vi "Sweep_AIWFM_time.vi"(8 "error in (no error)":errorcluster, 11 "Transport":refnum<class "SMO.Transport.lvclass">) -> (0 "error out":errorcluster, 3 "Transport.lvclass":refnum<class "SMO.Transport.lvclass">)   [LabVIEW 2019, in "SMO.Transport.lvclass"]
uses:
  SMO.Transport.lvclass
  <userlib>/LevyLab/Instrument Framework/Instrument Types/Cryostat/Instrument.Cryostat.lvclass
  SMO.Control Experiment/SMO.Control Experiment.lvclass
  <userlib>/LevyLab/Lockin-Multichannel/Instrument.Lockin/Instrument.Lockin.lvclass
  <userlib>/LevyLab/Krohn Hite 7008/Instrument.KH7008.lvclass
  SMO.Control Experiment/Private/Control Experiment SM/Typedefs/Instruments--cluster.ctl
  <userlib>/LevyLab/Instrument Framework/Instrument Types/VSource/Instrument.VSource.lvclass
  <userlib>/LevyLab/Instrument Framework/Instrument Types/VNA/Instrument.VNA.lvclass
  <userlib>/LevyLab/Instrument Framework/Instrument Types/Strain/Instrument.Strain.lvclass
  <userlib>/LevyLab/Instrument Framework/Instrument Types/CBridge/Instrument.CBridge.lvclass
  <vilib>/Waveform/WDTOps.llb/WDT Append Waveforms DBL.vi
  <userlib>/LevyLab/XY Utilities/xy_utilities.lvlib
  <userlib>/LevyLab/XY Utilities/subVIs/Waveform to XY (single).vi
  <userlib>/LevyLab/XY Utilities/subVIs/Get X and Y (single).vi
  <userlib>/LevyLab/Lockin-Multichannel/Lockin.DAQ/Typedefs/State-enum.ctl
  <userlib>/LevyLab/Lockin-Multichannel/Lockin.DAQ/Typedefs/Sweep Configuration--Cluster.ctl
  <userlib>/LevyLab/Lockin-Multichannel/Lockin.DAQ/Typedefs/Sweep Pattern--Enum.ctl
  <userlib>/LevyLab/Lockin-Multichannel/Instrument.Lockinl.UI/Typedefs/Sweep Channel--Cluster.ctl
  <userlib>/LevyLab/Instrument Framework/Instrument Types/Delay Line/Instrument.DelayLine.lvclass
panel:
  out "elapsed time (s)":u32=36594
  out "time b/w points (ms)":u32=533
  in  "Stop":bool
  in  "Tab Control":enum32{"Control", "Waveform", "Other"}(tab)
  in  "Sweep Time (s)":dbl=10.0 format="%#_3p"
  in  "Initial Wait (s)":u32=1
  in  "Return to Start":bool=TRUE
  in  "wait (ms)":u32=500
  in  "Experiment Description":string="SA40321H:\nT=80mK, BG=0V, B=-9T\nLoop 0: sgR: -1V to 1V, 20mV step\nInner loop: I+/I-: 28/2   -180mV to 220mV, sweep time 10s\nsgL (lead 1): 0V\nsgR (lead 3): sweep\n    \nI+/I-: 28/2   -180mV to 220mV, sweep time 10s\nV+/V-: 5/2\nsgL-lead 1; sgR-lead 3\n\ntc: 100ms\norder: 4\n\n"
  in  "Experiment Folder":string="01-sgR IV for RD"
  in  "Channels":T1[](array[typedef]) {"Channel" items=["AO1"=1, "AO2"=2]; "Start" format="%#_6p"; "End" format="%#_6p"}
  out "AO":waveform(dbl)(graph)={"t0"=timestamp(3666661573.979815 s since 1904-01-01), "dt"=0.0009999999996825864, "Y"=array[14000 elements]}
  out "AI vs AO":cluster{"Y":dbl[], "Y":dbl[]}[](graph)
  out "AI":waveform(dbl)[](graph)=[{"t0"=timestamp(3666661571.9305677 s since 1904-01-01), "dt"=0.0009999999996825864, "Y"=array[14000 elements], "attributes"=variant("NI_ChannelName"=variant(string "Dev1/ai0"), "NI_UnitDescription"=variant(string "Volts"))}, {"t0"=timestamp(3666661571.9305677 s since 1904-01-01), "dt"=0.0009999999996825864, "Y"=array[14000 elements], "attributes"=variant("NI_ChannelName"=variant(string "Dev1/ai1"), "NI_UnitDescription"=variant(string "Volts"))}, {"t0"=timestamp(3666661571.9305677 s since 1904-01-01), "dt"=0.0009999999996825864, "Y"=array[14000 elements], "attributes"=variant("NI_ChannelName"=variant(string "PXI1Slot8/ai0"), "NI_UnitDescription"=variant(string "Volts"))}, {"t0"=timestamp(3666661571.9305677 s since 1904-01-01), "dt"=0.0009999999996825864, "Y"=array[14000 elements], "attributes"=variant("NI_ChannelName"=variant(string "PXI1Slot8/ai1"), "NI_UnitDescription"=variant(string "Volts"))}, {"t0"=timestamp(3666661569.527568 s since 1904-01-01), "dt"=0.0009999999996825864, "Y"=array[14000 elements], "attributes"=variant("NI_ChannelName"=variant(string "Dev2/ai0"), "NI_UnitDescription"=variant(string "Volts"))}, {"t0"=timestamp(3666661569.527568 s since 1904-01-01), "dt"=0.0009999999996825864, "Y"=array[14000 elements], "attributes"=variant("NI_ChannelName"=variant(string "Dev2/ai1"), "NI_UnitDescription"=variant(string "Volts"))}]
  out "Status":T3
  out "Current State":string="File: Save"
  # "*** These controls are only read if this VI is the top level. If is is called from Sweep Control then the folder and comments come from Sweep Control.vi ***"
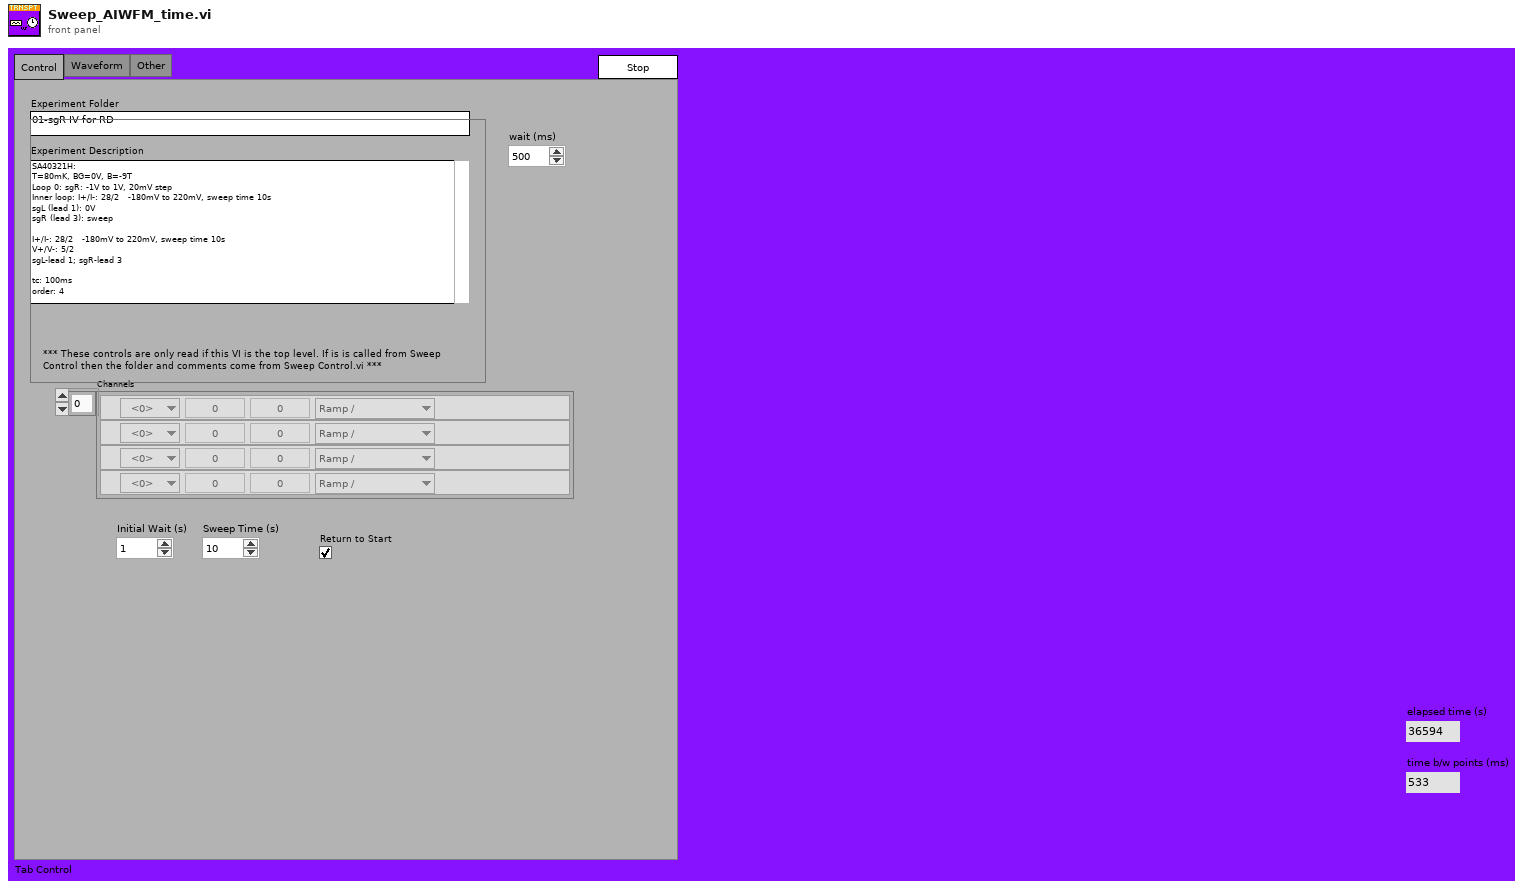
[diagram p1: front panel]
types:
  T1 = typedef "Instrument.Lockin.UI.lvclass/Sweep Channel--Cluster.ctl" = cluster{"End":dbl, "Start":dbl, "Channel":u16, "Pattern":T2}
  T2 = typedef "Lockin.DAQ.lvclass/Sweep Pattern--Enum.ctl" = enum16{"Ramp /", "Ramp /\\", "Smooth Ramp _/", "Smooth Ramp _/\\_", "Frequency"}
  T3 = typedef "Lockin.DAQ.lvclass/State-enum.ctl" = enum16{"idle", "created", "started", "stopped", "sweeping"}
  T4 = enum32{"Invalid", "Standard", "Closed", "Hidden", "Minimized", "Maximized"}
  T5 = enum32{"invalid app kind", "Development System", "Run Time System", "Student Edition", "Embedded LabVIEW", "Evaluation", "Custom"}
  T6 = typedef "SMO.Control Experiment.lvclass/Instruments--cluster.ctl" = cluster{"Lockin":refnum<class "Instrument.Lockin.lvclass">, "Temperature":refnum<class "Instrument.Cryostat.lvclass">, "Magnet":refnum<class "Instrument.Cryostat.lvclass">, "Rotator":refnum<class "Instrument.Cryostat.lvclass">, "Level":refnum<class "Instrument.Cryostat.lvclass">, "C Bridge":refnum<class "Instrument.CBridge.lvclass">, "Optical Delay Line":refnum<class "Instrument.DelayLine.lvclass">, "Strain Cell":refnum<class "Instrument.Strain.lvclass">, "VNA":refnum<class "Instrument.VNA.lvclass">, "Voltage Source":refnum<class "Instrument.VSource.lvclass">, "KH7008":refnum<class "Instrument.KH7008.lvclass">[]}
  T7 = typedef "Lockin.DAQ.lvclass/Sweep Configuration--Cluster.ctl" = cluster{"Sweep Time (s)":dbl, "Initial Wait (s)":dbl, "Return to Start":bool, "Channels":T1[]}
  T8 = cluster{"Core":cluster{"Current VI Reference":refnum<vi>, "Close Panel on Exit?":bool}, "Transport":refnum<class "SMO.Transport.lvclass">, "Control Experiment":refnum<class "SMO.Control Experiment.lvclass">, "Notifier":refnum<notifier>, "Instruments":T6, "path":path, "time":dbl, "temperature":dbl, "magnet field":dbl, "AI XY (new)":cluster{dbl[], dbl[]}[], "AI XY (all)":cluster{dbl[], dbl[]}[], "AI Waveform (s)":waveform(dbl)[], "t0":timestamp, "ms [0]":u32, "ms [i]":u32, "AO Waveform (s)":waveform(dbl)[], "Execution:State":enum32{"Bad", "Idle", "Run top level", "Running"}}
  T9 = enum32{"Bad", "Idle", "Run top level", "Running"}
  T10 = cluster{"Current VI Reference":refnum<vi>, "Close Panel on Exit?":bool}
  T11 = typedef "Instrument.DAQ.lvclass/Get State-enum.ctl" = enum16{"idle", "created", "started", "stopped", "sweeping"}
  T12 = typedef "Instrument.DAQ.lvclass/AO.Channel--Cluster--Array.ctl" = T13[]
  T13 = typedef "Instrument.DAQ.lvclass/AO.Channel--Cluster.ctl" = cluster{"Enable?":bool, "Channel":i32, "Amplitude":dbl, "Offset":dbl, "Frequency":dbl, "Phase":dbl, "Function":T14, "Sweeping?":bool}
  T14 = typedef "Instrument.DAQ.lvclass/AO.Channel.Function--Enum.ctl" = enum16{"Sine", "Triangle", "Square"}
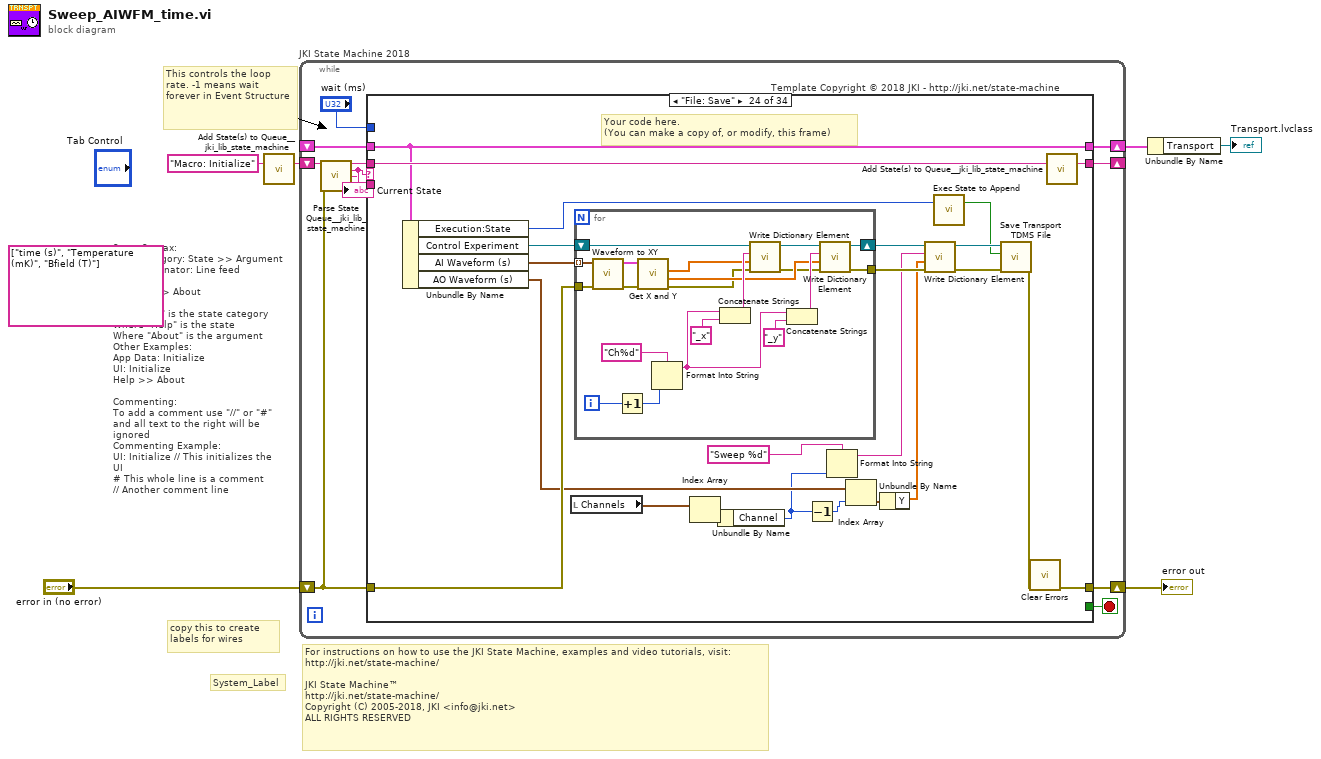
[diagram p0: block diagram]
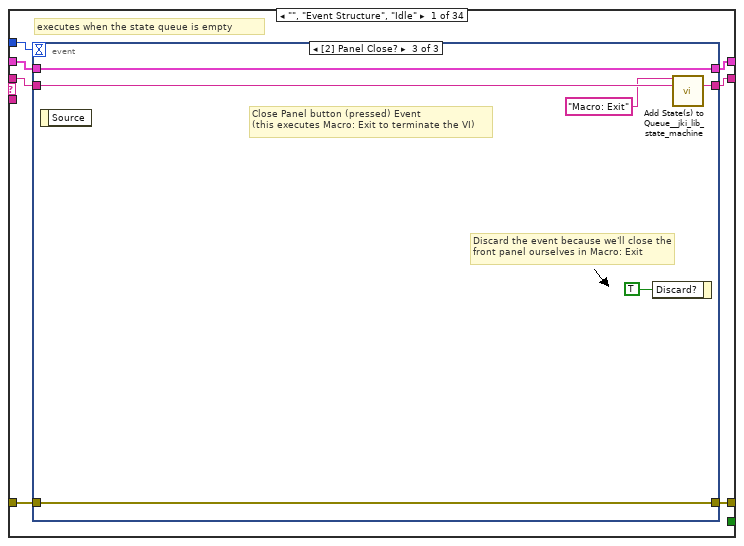
[diagram p2: hidden frame]
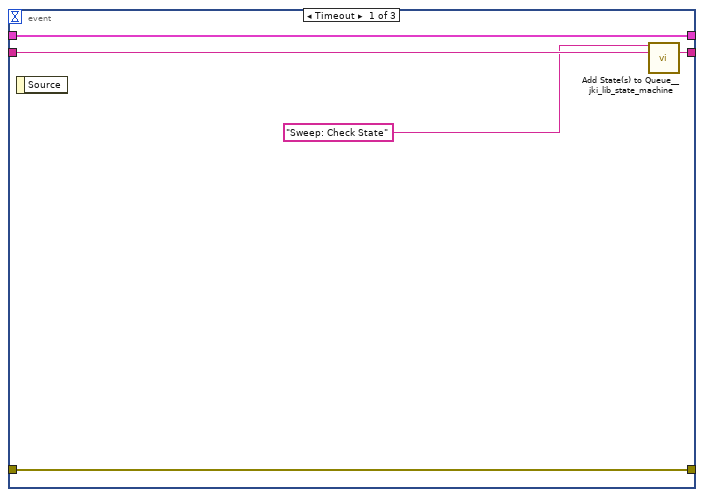
[diagram p3: hidden frame]
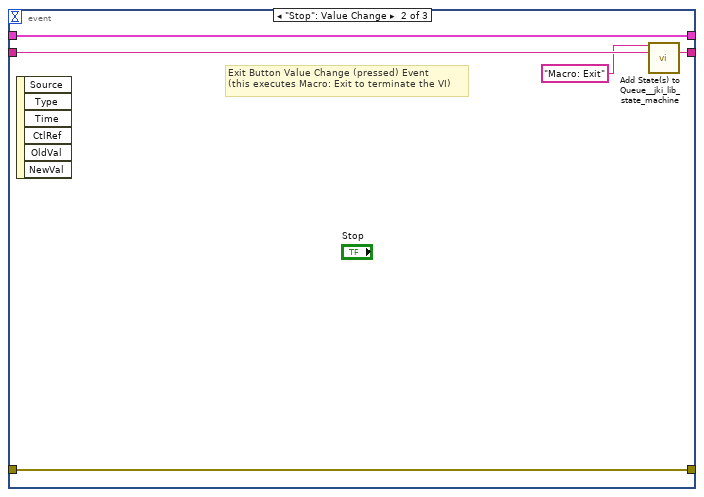
[diagram p4: hidden frame]
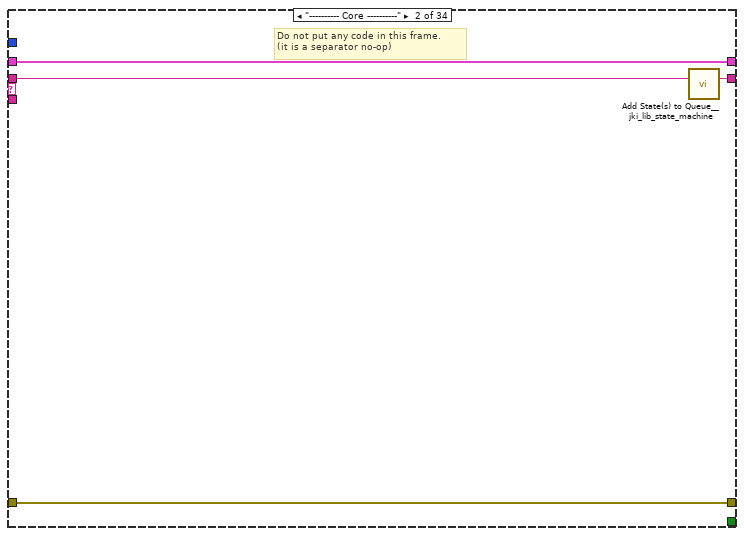
[diagram p5: hidden frame]
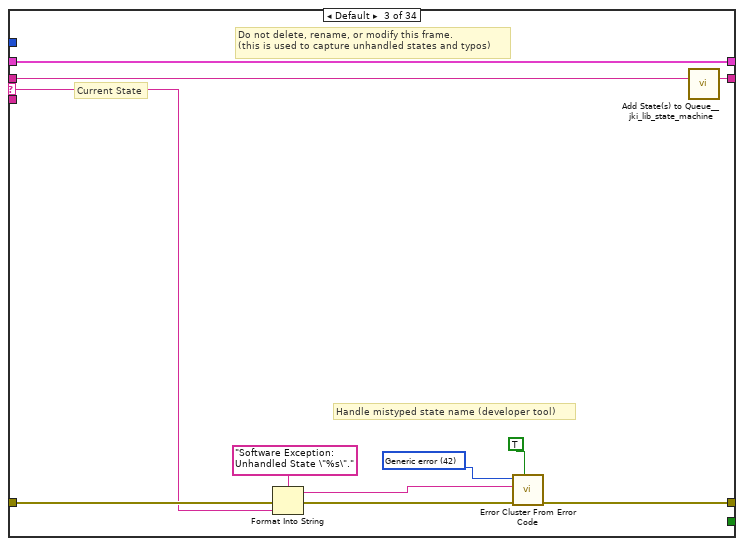
[diagram p6: hidden frame]
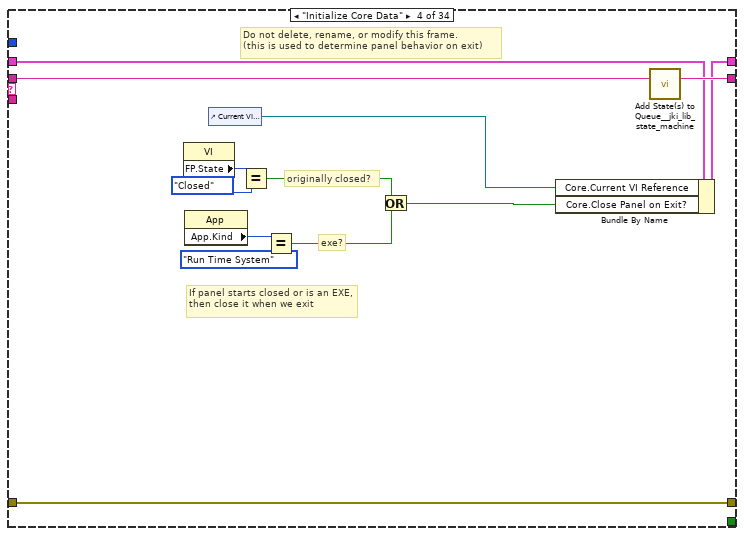
[diagram p7: hidden frame]
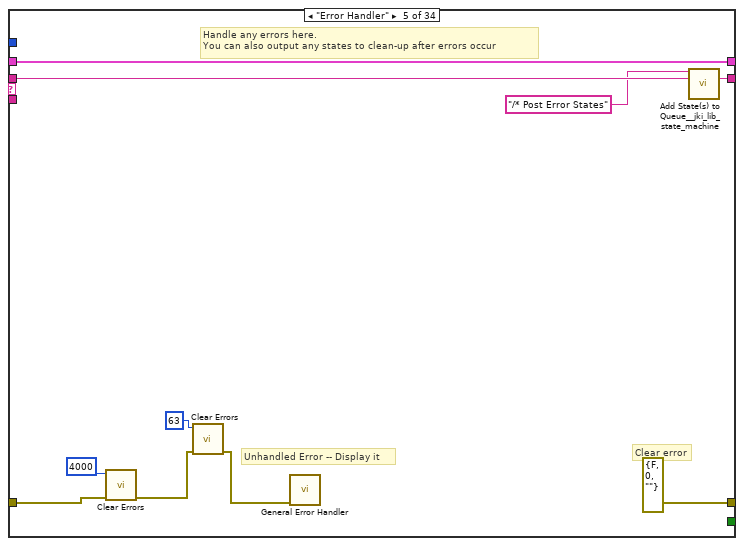
[diagram p8: hidden frame]
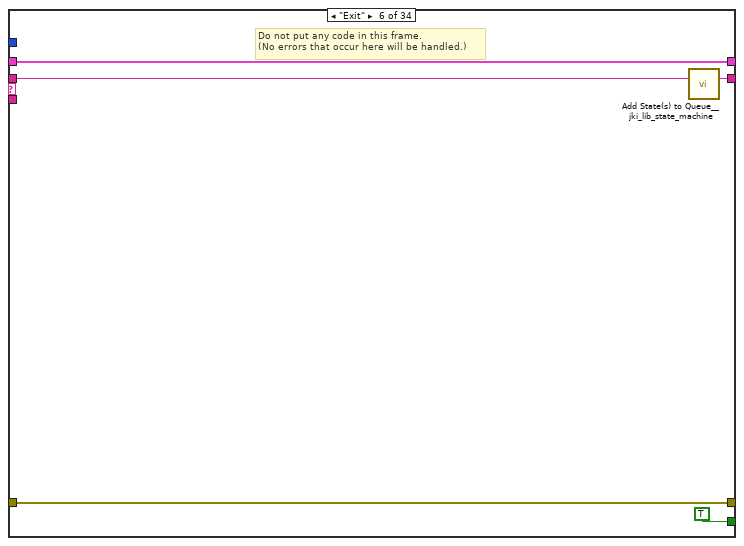
[diagram p9: hidden frame]
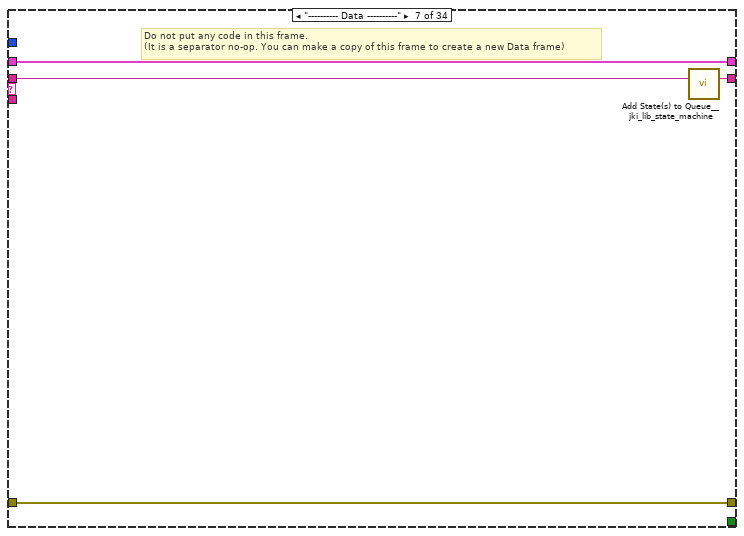
[diagram p10: hidden frame]
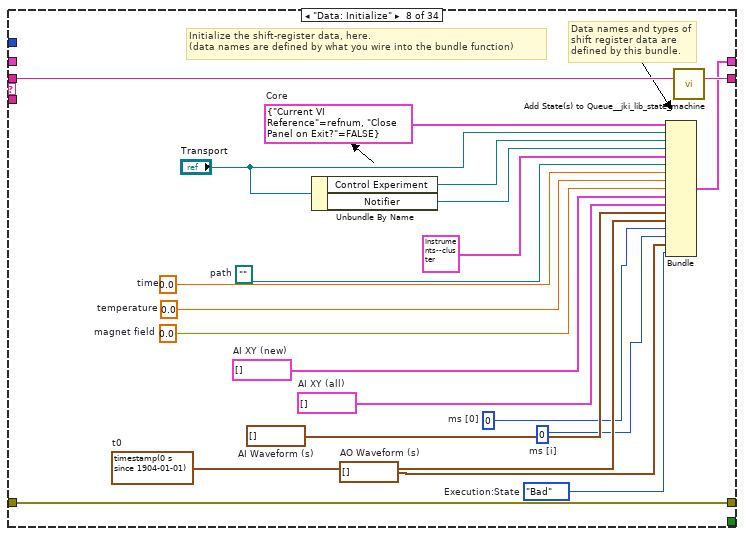
[diagram p11: hidden frame]
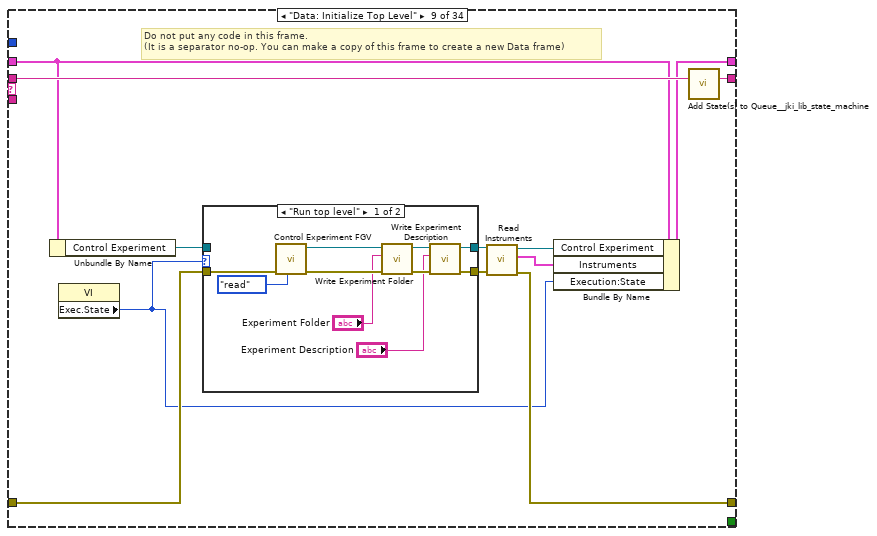
[diagram p12: hidden frame]
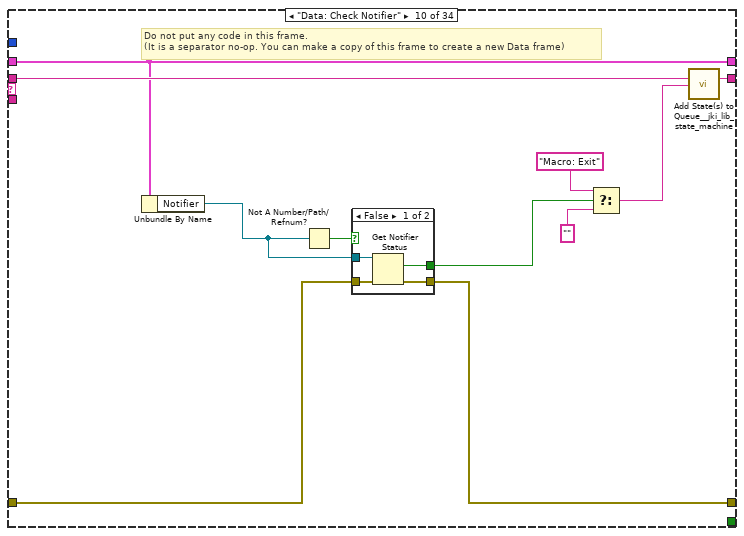
[diagram p14: hidden frame]
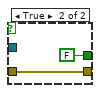
[diagram p15: hidden frame]
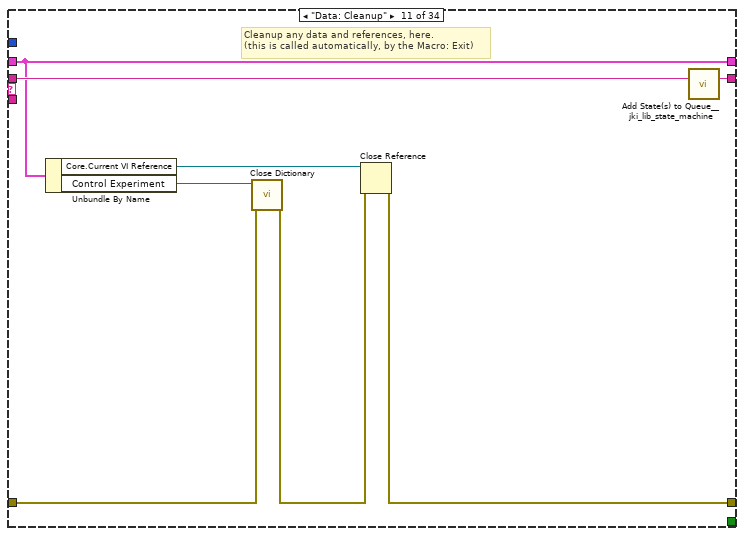
[diagram p16: hidden frame]
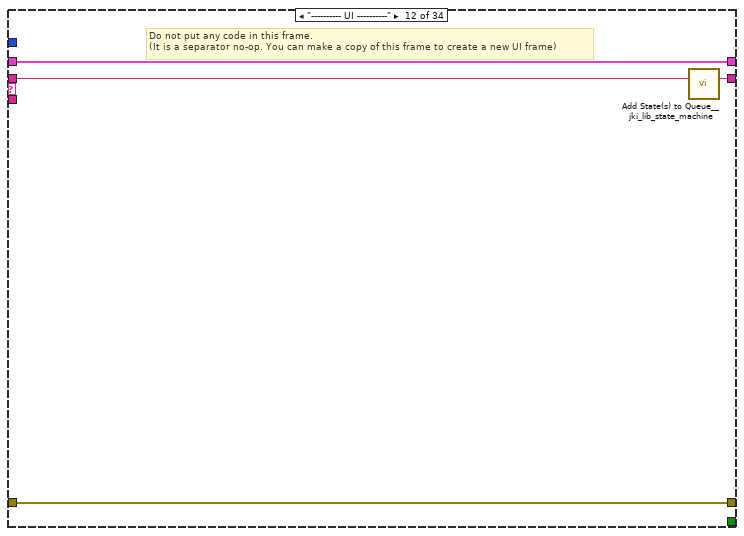
[diagram p17: hidden frame]
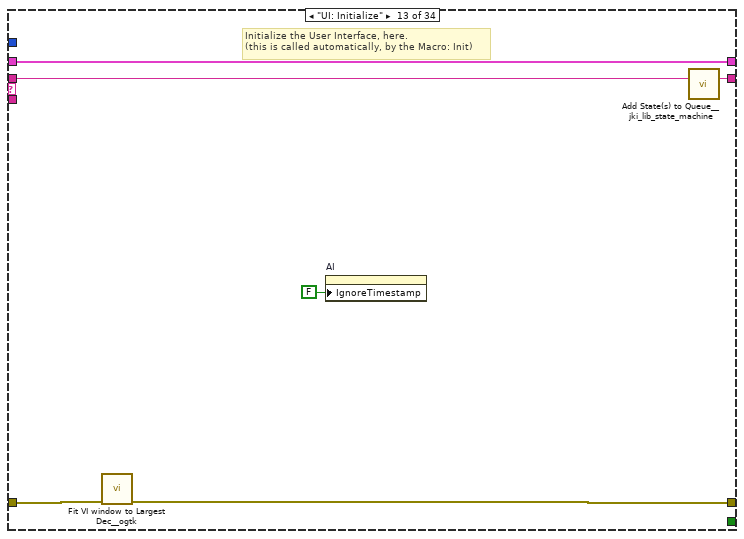
[diagram p18: hidden frame]
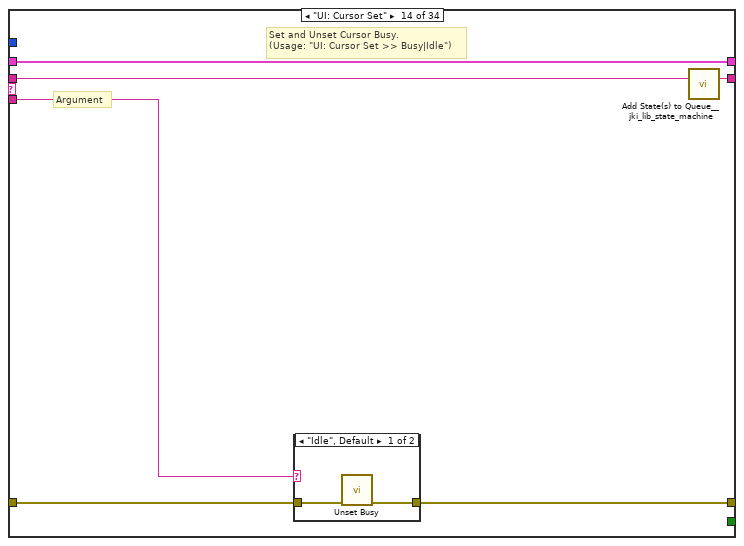
[diagram p19: hidden frame]
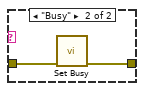
[diagram p20: hidden frame]
diagram:
  (unwired) string[] ["time (s)", "Temperature (mK)", "Bfield (T)"] ("wavenames (.Vx, etc)")
  # "For instructions on how to use the JKI State Machine, examples and video tutorials, visit:\nhttp://jki.net/state-machine/\n\nJKI State Machine™\nhttp://jki.net/state-machine/\nCopyright (C) 2005-2018, JKI <info@jki.net>\nALL RIGHTS RESERVED"
  # "State Syntax:\nStateCategory: State >> Argument\nLine Terminator: Line feed\nExample:\nUI: Help >> About\n\nWhere \"UI\" is the state category\nWhere \"Help\" is the state\nWhere \"About\" is the argument\nOther Examples:\nApp Data: Initialize\nUI: Initialize\nHelp >> About\n\nCommenting:\nTo add a comment use \"//\" or \"#\" and all text to the right will be ignored\nCommenting Example:\nUI: Initialize // This initializes the UI\n# This whole line is a comment\n// Another comment line"
  # "copy this to create labels for wires"
  # "This controls the loop rate. -1 means wait forever in Event Structure"
  # "System_Label"
  n1 = call <vilib>:"Add State(s) to Queue__jki_lib_state_machine.vi"("State(s) in (\"\")"="Macro: Initialize") -> ("States Out"=w6:string)  [unwired: 14 in]
  n2 = while "JKI State Machine 2018" {
    shift-right: [w10] -> w2
    shift-left: _ -> [w9]
    shift-right: [w13] -> w3
    shift-left: "error in (no error)" -> [w8]
    shift-right: [w12] -> _
    shift-left: w6 -> [w14]
    stop <- w11 stop-if-true
    # "Template Copyright © 2018 JKI - http://jki.net/state-machine"
    n3 = call <vilib>:"Parse State Queue__jki_lib_state_machine.vi"("State Queue"=w14, "Error In (no error)"=w8) -> ("Remaining States"=w16:string, "Current State"=w17:string, "Arguments"=w15:string)  [unwired: 11 in]
    "Current State" <- w17
    n4 = case shown="\"File: Save\"" w17 {
      selector: w17 -> [_ _ w45 _ _ _ _ _ _ _ _ _ _ _ _ _ _ _ _ _ _ _ _ _ _ _ _ _ _ _ _ _ _ _]
      tunnel: w16 -> [w24 w44 w49 w68 w78 w83 w87 w108 w120 w143 w157 w161 w167 w173 w184 w261 w279 w283 w288 w293 w301 w311 w315 w338 w362 w374 w382 w397 w405 w411 w422 w434 w446 w460]
      tunnel: w15 -> [_ _ _ _ _ _ _ _ _ _ _ _ _ w168 w178 _ _ _ _ _ _ _ _ _ _ _ _ _ _ _ _ _ _ _]
      tunnel: w9 -> [w22 w41 w47 w61 w75 w81 w84 _ w116 w140 w153 w158 w165 w171 w180 w259 w270 w280 w285 w290 w298 w308 w312 w336 w359 w372 w377 w394 w398 w408 w418 w430 w444 w457]
      tunnel: [w21 w42 w51 w65 errorcluster {"status"=FALSE, "code"=0, "source"=""} ("error out") w80 w85 w105 w110 w138 w154 w159 w163 w169 w181 w258 w267 w281 w286 w291 w299 w309 w313 w335 w360 w369 w375 w392 w400 w409 w412 w423 w439 w451] -> w13
      tunnel: w8 -> [w20 w42 w50 w65 w72 w80 w85 w105 w115 w137 w151 w159 w164 w170 w182 w258 w268 w281 w286 w291 w299 w309 w313 w331 w360 w370 w376 w393 w401 w409 w415 w431 w438 w452]
      tunnel: [w23 w43 w48 w67 w77 w82 w86 w107 w119 w142 w156 w160 w166 w172 w183 w260 w278 w282 w287 w292 w300 w310 w314 w337 w361 w373 w381 w396 w404 w410 w421 w433 w445 w459] -> w12
      tunnel: [_ _ _ _ _ TRUE _ _ _ _ _ _ _ _ _ _ _ _ _ _ _ _ _ _ _ _ _ _ _ _ _ _ _ _] -> w11
      tunnel: [w19 w41 w47 w66 w75 w81 w84 w106 w117 w140 w153 w158 w165 w171 w180 w259 w269 w280 w285 w290 w298 w308 w312 w336 w359 w372 w377 w394 w398 w408 w419 w429 w443 w458] -> w10
      tunnel: "wait (ms)" -> [w18 _ _ _ _ _ _ _ _ _ _ _ _ _ _ _ _ _ _ _ _ _ _ _ _ _ _ _ _ _ _ _ _ _]
      frame "", "Event Structure", "Idle" {
        # "executes when the state queue is empty"
        n5 = event shown="[2] Panel Close?" {
          selector: _ -> [_ _ _]
          dyn-events: _ -> [_ _ _]
          timeout: w18 -> [_ _ _]
          tunnel: w24 -> [w29 w34 w40]
          tunnel: [w28 w33 w39] -> w23
          tunnel: w22 -> [w26 w31 w37]
          tunnel: [w27 w32 w38] -> w21
          tunnel: w20 -> [w27 w32 w38]
          tunnel: [w26 w31 w37] -> w19
          event Timeout {
            n6 = event-data() -> ()  [unwired: 1 in, 1 out]
            n7 = call <vilib>:"Add State(s) to Queue__jki_lib_state_machine.vi"("State(s) in Front (\"\")"="Sweep: Check State" ("State(s) in Front (\"\")"), "State(s) in (\"\")"=w29) -> ("States Out"=w28:string)  [unwired: 13 in]
          }
          event "Stop": Value Change {
            # "Exit Button Value Change (pressed) Event\n(this executes Macro: Exit to terminate the VI)"
            n8 = event-data() -> ()  [unwired: 1 in, 6 out]
            n9 = call <vilib>:"Add State(s) to Queue__jki_lib_state_machine.vi"("State(s) in Front (\"\")"="Macro: Exit", "State(s) in (\"\")"=w34) -> ("States Out"=w33:string)  [unwired: 13 in]
          }
          event Panel Close? {
            # "Discard the event because we'll close the front panel ourselves in Macro: Exit"
            # "Close Panel button (pressed) Event\n(this executes Macro: Exit to terminate the VI)"
            n10 = event-data() -> ()  [unwired: 1 in, 1 out]
            n11 = event-data("Discard?"=TRUE) -> ()  [unwired: 1 in, 1 out]
            n12 = call <vilib>:"Add State(s) to Queue__jki_lib_state_machine.vi"("State(s) in Front (\"\")"="Macro: Exit", "State(s) in (\"\")"=w40) -> ("States Out"=w39:string)  [unwired: 13 in]
          }
        }
      }
      frame "---------- Core ----------" {
        # "Do not put any code in this frame.\n(it is a separator no-op)"
        n13 = call <vilib>:"Add State(s) to Queue__jki_lib_state_machine.vi"("State(s) in (\"\")"=w44) -> ("States Out"=w43:string)  [unwired: 14 in]
      }
      frame Default {
        w54 = 42 items=["No error", "Argument error", "Memory is full", "Out of zone", "End of file", "File already open", "Generic file I/O error", "File not found", "File permission error", "Disk is full", "Duplicate path", "Too many files open", "System feature not enabled", "Resource file not found", "Cannot add resource", "Resource not found", "Image not found", "Image memory error", "Pen does not exist", "Config type invalid", "Config token not found", "Config parse error", "Config memory error", "Bad external code format", "Bad external code offset", "External code not present", "Null window", "Destroy window error", "Null menu", "Print aborted", "Bad print record", "Print driver error", "Windows error during printing", "Memory error during printing", "Print dialog error", "Generic print error", "Invalid device refnum", "Device not found", "Device parameter error", "Device unit error", "Cannot open device", "Device call aborted", "Generic error", "Cancelled by user", "Object ID too low", "Object ID too high", "Object not in heap", "Unknown heap", "Unknown object (invalid DefProc)", "Unknown object (DefProc not in table)", "Message out of range", "Invalid (null) method", "Unknown message", "Manager call not supported", "Bad address", "Network operation in progress", "Network operation timed out", "Connection is busy", "Network attribute not supported", "Network error", "Address in use", "System out of memory", "Connection aborted", "Connection refused", "Not connected", "Already connected", "Connection closed", "Initialization error (interapplication manager)", "Bad occurrence", "Wait on unbound occurrence handler", "Occurrence queue overflow", "Datalog type conflict", "Unused", "Unrecognized type (interapplication manager)", "Memory corrupt", "Failed to make temporary DLL", "Old CIN version", "Drag socket not found", "Failed to load drop-object", "Failed to register OLE object", "Failed to release OLE object", "Format specifier type mismatch", "Unknown format specifier", "Too few format specifiers", "Too many format specifiers", "Scan failed", "Newer CIN version", "Error converting to variant", "Runtime menu error", "Password tampered", "Variant attribute not found", "Incompatible variant data type", "Event data is not available", "Event Store is not present", "Occurrence is not found", "Event Queue is not created", "Event info is not available", "Refnum passed is NULL", "Error retrieving Class GUID", "Error retrieving CoClass GUID", "Error retrieving TypeLib GUID.", "Bad built application magic bytes.", "Specific driver is different from the specific driver associated with the Logical Name.", "There is no session opened to the class driver.", "Max Error", "MAX - Error with config objects", "MAX - Error loading configuration", "MAX - Group not supported"]
        # "Current State"
        # "Do not delete, rename, or modify this frame.\n(this is used to capture unhandled states and typos)"
        # "Handle mistyped state name (developer tool)"
        n14 = Format Into String(format string="Software Exception: Unhandled State \"%s\"." ("message"), error in=w50, w45) -> (resulting string=w53:string, error out=w52:errorcluster)  [unwired: 1 in]
        n15 = call <vilib>:"Error Cluster From Error Code.vi"("show call chain? (False)"=TRUE, "error in (no error)"=w52, "error message (\"\")"=w53, "error code (0)"=w54) -> ("error out"=w51:errorcluster)  [unwired: 5 in]
        n16 = call <vilib>:"Add State(s) to Queue__jki_lib_state_machine.vi"("State(s) in (\"\")"=w49) -> ("States Out"=w48:string)  [unwired: 14 in]
      }
      frame "Initialize Core Data" {
        # "Do not delete, rename, or modify this frame.\n(this is used to determine panel behavior on exit)"
        # "originally closed?"
        # "exe?"
        # "If panel starts closed or is an EXE, then close it when we exit"
        n17 = property class="VI"() -> ("FP.State"=w58:T4)  [unwired: 2 in, 2 out]
        n18 = property class="App"() -> ("App.Kind"=w64:T5)  [unwired: 2 in, 2 out]
        n19 = control-ref of="Current VI Reference"() -> (w59:refnum<vi>)
        n20 = Equal?(x=w58, y=T4."Closed" ("Front Panel Window:State")) -> (x = y?=w56:bool)
        n21 = Equal?(x=w64, y=T5."Run Time System" ("Application:Kind")) -> (x = y?=w62:bool)
        n22 = Or(x=w56, y=w62) -> (x .or. y?=w60:bool)
        n23 = Bundle By Name(cluster=w61, "Core.Current VI Reference"=w59, "Core.Close Panel on Exit?"=w60) -> (w66:T8)
        n24 = call <vilib>:"Add State(s) to Queue__jki_lib_state_machine.vi"("State(s) in (\"\")"=w68) -> ("States Out"=w67:string)  [unwired: 14 in]
      }
      frame "Error Handler" {
        # "Unhandled Error -- Display it"
        # "Handle any errors here.\nYou can also output any states to clean-up after errors occur"
        # "Clear error"
        n25 = call <vilib>:"Clear Errors.vi"("error in (no error)"=w72, "specific error code to clear (0: all)"=4000) -> ("error out"=w70:errorcluster)  [unwired: 4 in, 1 out]
        n26 = call <vilib>:"Clear Errors.vi"("error in (no error)"=w70, "specific error code to clear (0: all)"=63) -> ("error out"=w69:errorcluster)  [unwired: 4 in, 1 out]
        n27 = call <vilib>:"General Error Handler.vi"("error in (no error)"=w69) -> ()  [unwired: 10 in, 5 out]
        n28 = call <vilib>:"Add State(s) to Queue__jki_lib_state_machine.vi"("State(s) in Front (\"\")"="/* Post Error States", "State(s) in (\"\")"=w78) -> ("States Out"=w77:string)  [unwired: 13 in]
      }
      frame "Exit" {
        # "Do not put any code in this frame.\n(No errors that occur here will be handled.)"
        n29 = call <vilib>:"Add State(s) to Queue__jki_lib_state_machine.vi"("State(s) in (\"\")"=w83) -> ("States Out"=w82:string)  [unwired: 14 in]
      }
      frame "---------- Data ----------" {
        # "Do not put any code in this frame.\n(It is a separator no-op. You can make a copy of this frame to create a new Data frame)"
        n30 = call <vilib>:"Add State(s) to Queue__jki_lib_state_machine.vi"("State(s) in (\"\")"=w87) -> ("States Out"=w86:string)  [unwired: 14 in]
      }
      frame "Data: Initialize" {
        w88 = T9."Bad"  # Execution:State
        w89 = waveform(dbl)[] []  # AO Waveform (s)
        w90 = u32 0  # ms [i]
        w91 = u32 0  # ms [0]
        w92 = timestamp(0 s since 1904-01-01)  # t0
        w93 = waveform(dbl)[] []  # AI Waveform (s)
        w98 = cluster{dbl[], dbl[]}[] []  # AI XY (new)
        w99 = cluster{dbl[], dbl[]}[] []  # AI XY (all)
        w96 = 0.0  # magnet field
        w95 = 0.0  # temperature
        w94 = 0.0  # time
        w103 = path ""  # path
        w104 = T10 {"Current VI Reference"=refnum, "Close Panel on Exit?"=FALSE}  # Core
        # "Data names and types of shift register data are defined by this bundle."
        # "Initialize the shift-register data, here.\n(data names are defined by what you wire into the bundle function)"
        n31 = Unbundle By Name("Transport") -> ("Control Experiment"=w101:refnum<class "SMO.Control Experiment.lvclass">, "Notifier"=w100:refnum<notifier>)
        n32 = Bundle("Core"=w104, "Transport"="Transport", "Control Experiment"=w101, "Notifier"=w100, "Instruments"=T6 {"Lockin"=refnum, "Temperature"=refnum, "Magnet"=refnum, "Rotator"=refnum, "Level"=refnum, "C Bridge"=refnum, "Optical Delay Line"=refnum, "Strain Cell"=refnum, "VNA"=refnum, "Voltage Source"=refnum, "KH7008"=[]}, "path"=w103, "time"=w94, "temperature"=w95, "magnet field"=w96, "AI XY (new)"=w98, "AI XY (all)"=w99, "AI Waveform (s)"=w93, "t0"=w92, "ms [0]"=w91, "ms [i]"=w90, "AO Waveform (s)"=w89, "Execution:State"=w88) -> (w106:T8)  [unwired: 1 in]
        n33 = call <vilib>:"Add State(s) to Queue__jki_lib_state_machine.vi"("State(s) in (\"\")"=w108) -> ("States Out"=w107:string)  [unwired: 14 in]
      }
      frame "Data: Initialize Top Level" {
        # "Do not put any code in this frame.\n(It is a separator no-op. You can make a copy of this frame to create a new Data frame)"
        n34 = Unbundle By Name(w116) -> ("Control Experiment"=w118:refnum<class "SMO.Control Experiment.lvclass">)
        n35 = property class="VI"() -> ("Exec.State"=w109:T9)  [unwired: 2 in, 2 out]
        n36 = case shown="\"Run top level\"" w109 {
          tunnel: w115 -> [w130 w131]
          tunnel: [w125 w131] -> w114
          tunnel: [w124 w132] -> w113
          tunnel: w118 -> [_ w132]
          frame "Run top level" {
            n37 = call "Control Experiment FGV.vi"("Function"=enum16{"read", "write"}."read", "error in (no error)"=w130) -> ("error out"=w128:errorcluster, "Control Experiment out"=w129:refnum<class "SMO.Control Experiment.lvclass">)  [unwired: 8 in]
            n38 = call "Write Experiment Folder.vi"("error in (no error)"=w128, "Experiment Folder"="Experiment Folder", "Control Experiment"=w129) -> ("error out"=w126:errorcluster, "Control Experiment out"=w127:refnum<class "SMO.Control Experiment.lvclass">)  [unwired: 7 in]
            n39 = call "Write Experiment Description.vi"("error in (no error)"=w126, "Experiment Description"="Experiment Description", "Control Experiment"=w127) -> ("error out"=w125:errorcluster, "Control Experiment out"=w124:refnum<class "SMO.Control Experiment.lvclass">)  [unwired: 7 in]
          }
          frame "Running", Default {
          }
        }
        n40 = call "Read Instruments.vi"("error in (no error)"=w114, "Control Experiment"=w113) -> ("error out"=w110:errorcluster, "Instruments"=w111:T6, "Control Experiment out"=w112:refnum<class "SMO.Control Experiment.lvclass">)  [unwired: 7 in]
        n41 = Bundle By Name(cluster=w116, "Control Experiment"=w112, "Instruments"=w111, "Execution:State"=w109) -> (w117:T8)
        n42 = call <vilib>:"Add State(s) to Queue__jki_lib_state_machine.vi"("State(s) in (\"\")"=w120) -> ("States Out"=w119:string)  [unwired: 14 in]
      }
      frame "Data: Check Notifier" {
        # "Do not put any code in this frame.\n(It is a separator no-op. You can make a copy of this frame to create a new Data frame)"
        n43 = Unbundle By Name(w140) -> ("Notifier"=w139:refnum<notifier>)
        n44 = Not A Number/Path/Refnum?(number/path/refnum=w139) -> (NaN/Path/Refnum?=w141:bool)
        n45 = case shown="False" w141 {
          tunnel: [w147 FALSE] -> w136
          tunnel: [w146 w148] -> w138
          tunnel: w139 -> [w145 _]
          tunnel: w137 -> [w144 w148]
          frame False {
            n46 = Get Notifier Status(notifier=w145, error in (no error)=w144) -> (current notification=w147:bool, error out=w146:errorcluster)  [unwired: 3 out]
          }
          frame True {
          }
        }
        n47 = Select(t="Macro: Exit", s=w136, f="") -> (s? t:f=w133:string)
        n48 = call <vilib>:"Add State(s) to Queue__jki_lib_state_machine.vi"("State(s) in (\"\")"=w143, "State(s) at Back (\"\")"=w133) -> ("States Out"=w142:string)  [unwired: 13 in]
      }
      frame "Data: Cleanup" {
        # "Cleanup any data and references, here.\n(this is called automatically, by the Macro: Exit)"
        n49 = Unbundle By Name(w153) -> ("Core.Current VI Reference"=w155:refnum<vi>, "Control Experiment"=w152:refnum<class "SMO.Control Experiment.lvclass">)
        n50 = call "Close Dictionary.vi"("error in (no error)"=w151, "Control Experiment"=w152) -> ("error out"=w150:errorcluster)  [unwired: 8 in, 1 out]
        n51 = Close Reference(reference=w155, error in (no error)=w150) -> (error out=w154:errorcluster)
        n52 = call <vilib>:"Add State(s) to Queue__jki_lib_state_machine.vi"("State(s) in (\"\")"=w157) -> ("States Out"=w156:string)  [unwired: 14 in]
      }
      frame "---------- UI ----------" {
        # "Do not put any code in this frame.\n(It is a separator no-op. You can make a copy of this frame to create a new UI frame)"
        n53 = call <vilib>:"Add State(s) to Queue__jki_lib_state_machine.vi"("State(s) in (\"\")"=w161) -> ("States Out"=w160:string)  [unwired: 14 in]
      }
      frame "UI: Initialize" {
        # "Initialize the User Interface, here.\n(this is called automatically, by the Macro: Init)"
        n54 = call <userlib>:"Fit VI window to Largest Dec__ogtk.vi"("error in (no error)"=w164) -> ("error out"=w163:errorcluster)  [unwired: 5 in, 1 out]
        n55 = property on="AI" class="WFGraph (strict)"("IgnoreTimestamp"=FALSE ("Ignore Timestamp")) -> ()  [unwired: 2 in, 2 out]
        n56 = call <vilib>:"Add State(s) to Queue__jki_lib_state_machine.vi"("State(s) in (\"\")"=w167) -> ("States Out"=w166:string)  [unwired: 14 in]
      }
      frame "UI: Cursor Set" {
        # "Argument"
        # "Set and Unset Cursor Busy.\n(Usage: \"UI: Cursor Set >> Busy|Idle\")"
        n57 = case shown="\"Idle\", Default" w168 {
          tunnel: w170 -> [w175 w177]
          tunnel: [w174 w176] -> w169
          frame "Idle", Default {
            n58 = call <vilib>:"Unset Busy.vi"("error in (no error)"=w175) -> ("error out"=w174:errorcluster)  [unwired: 10 in]
          }
          frame "Busy" {
            n59 = call <vilib>:"Set Busy.vi"("error in (no error)"=w177) -> ("error out"=w176:errorcluster)  [unwired: 9 in, 1 out]
          }
        }
        n60 = call <vilib>:"Add State(s) to Queue__jki_lib_state_machine.vi"("State(s) in (\"\")"=w173) -> ("States Out"=w172:string)  [unwired: 14 in]
      }
      frame "UI: Front Panel State" {
        # "Argument"
        # "Set Front Panel Open or Closed\n(Usage: \"UI: Front Panel State >> Open|Close\")"
        n61 = Unbundle By Name(w180) -> ("Core.Current VI Reference"=w179:refnum<vi>)
        n62 = case shown="\"Minimize\", \"Minimized\"" w178 {
          tunnel: w182 -> [w190 w205 w216 w229 w242]
          tunnel: [w192 w206 w218 w231 w244] -> w181
          tunnel: w179 -> [w191 w203 w217 w230 w243]
          frame "Open", "Standard", Default {
            w185 = T4."Standard" ("State")
            n63 = property class="VI"(reference=w191, error in=w190) -> (reference out=w188:refnum<vi>, error out=w189:errorcluster, "FP.State"=w187:T4)
            n64 = Not Equal?(x=w187, y=w185) -> (x != y?=w186:bool)
            n65 = case shown="True" w186 {
              tunnel: [w196 w198] -> w192
              tunnel: w189 -> [w195 w198]
              tunnel: w188 -> [w194 _]
              tunnel: w185 -> [w193 _]
              frame True {
                n66 = invoke class="VI" method="FP.Open"(reference=w194, error in=w195, "Activate"=TRUE, "State"=w193) -> (error out=w196:errorcluster)  [unwired: 1 in, 4 out]
              }
              frame False {
              }
            }
          }
          frame "Close", "Closed" {
            n67 = property class="VI"(reference=w203, error in=w205) -> (reference out=w202:refnum<vi>, error out=w204:errorcluster, "FP.State"=w200:T4)
            n68 = Not Equal?(x=w200, y=T4."Closed" ("Front Panel Window:State")) -> (x != y?=w199:bool)
            n69 = case shown="True" w199 {
              tunnel: [w207 w210] -> w206
              tunnel: w204 -> [w207 w209]
              tunnel: w202 -> [_ w208]
              frame False {
              }
              frame True {
                n70 = invoke class="VI" method="FP.Close"(reference=w208, error in=w209) -> (error out=w210:errorcluster)  [unwired: 1 in, 2 out]
              }
            }
          }
          frame "Hidden", "Hide" {
            w211 = T4."Hidden" ("State")
            n71 = property class="VI"(reference=w217, error in=w216) -> (reference out=w214:refnum<vi>, error out=w215:errorcluster, "FP.State"=w213:T4)
            n72 = Not Equal?(x=w213, y=w211) -> (x != y?=w212:bool)
            n73 = case shown="True" w212 {
              tunnel: [w222 w223] -> w218
              tunnel: w215 -> [w221 w223]
              tunnel: w214 -> [w220 _]
              tunnel: w211 -> [w219 _]
              frame True {
                n74 = invoke class="VI" method="FP.Open"(reference=w220, error in=w221, "State"=w219) -> (error out=w222:errorcluster)  [unwired: 2 in, 4 out]
              }
              frame False {
              }
            }
          }
          frame "Minimize", "Minimized" {
            w224 = T4."Minimized" ("State")
            n75 = property class="VI"(reference=w230, error in=w229) -> (reference out=w227:refnum<vi>, error out=w228:errorcluster, "FP.State"=w226:T4)
            n76 = Not Equal?(x=w226, y=w224) -> (x != y?=w225:bool)
            n77 = case shown="True" w225 {
              tunnel: [w235 w236] -> w231
              tunnel: w228 -> [w234 w236]
              tunnel: w227 -> [w233 _]
              tunnel: w224 -> [w232 _]
              frame True {
                n78 = invoke class="VI" method="FP.Open"(reference=w233, error in=w234, "State"=w232) -> (error out=w235:errorcluster)  [unwired: 2 in, 4 out]
              }
              frame False {
              }
            }
          }
          frame "Maximize", "Maximized" {
            w237 = T4."Maximized" ("State")
            n79 = property class="VI"(reference=w243, error in=w242) -> (reference out=w240:refnum<vi>, error out=w241:errorcluster, "FP.State"=w239:T4)
            n80 = Not Equal?(x=w239, y=w237) -> (x != y?=w238:bool)
            n81 = case shown="True" w238 {
              tunnel: [w248 w249] -> w244
              tunnel: w241 -> [w247 w249]
              tunnel: w240 -> [w246 _]
              tunnel: w237 -> [w245 _]
              frame True {
                n82 = invoke class="VI" method="FP.Open"(reference=w246, error in=w247, "State"=w245) -> (error out=w248:errorcluster)  [unwired: 2 in, 4 out]
              }
              frame False {
              }
            }
          }
        }
        n83 = call <vilib>:"Add State(s) to Queue__jki_lib_state_machine.vi"("State(s) in (\"\")"=w184) -> ("States Out"=w183:string)  [unwired: 14 in]
      }
      frame "UI: Update Graphs" {
        # "Do not put any code in this frame.\n(It is a separator no-op. You can make a copy of this frame to create a new UI frame)"
        n84 = local read "Channels"() -> (w255:T1[])
        n85 = Index Array(array=w255) -> (element=w254:T1)  [unwired: 1 in]
        n86 = Unbundle By Name(w259) -> ("AI Waveform (s)"=w257:waveform(dbl)[], "AO Waveform (s)"=w256:waveform(dbl)[])
        "AI" <- w257
        n87 = Unbundle By Name(w254) -> ("Channel"=w250:u16)
        n88 = Decrement(x=w250) -> (x-1=w253:u16)
        n89 = Index Array(array=w256, index=w253) -> (element=w251:waveform(dbl))
        "AO" <- w251
        n90 = for {
          tunnel: w257 -> [w266] mode=indexing
          tunnel: w251 -> [w265]
          tunnel: [w262] -> w252 mode=indexing
          n91 = Unbundle By Name(w265) -> ("Y"=w263:dbl[])
          n92 = Unbundle By Name(w266) -> ("Y"=w264:dbl[])
          n93 = Bundle("Y"=w263, "Y"=w264) -> (w262:cluster{"Y":dbl[], "Y":dbl[]})  [unwired: 1 in]
        }
        "AI vs AO" <- w252
        n94 = call <vilib>:"Add State(s) to Queue__jki_lib_state_machine.vi"("State(s) in (\"\")"=w261) -> ("States Out"=w260:string)  [unwired: 14 in]
      }
      frame "UI: Update Timer" {
        # "Do not put any code in this frame.\n(It is a separator no-op. You can make a copy of this frame to create a new UI frame)"
        n95 = Unbundle By Name(w270) -> ("ms [0]"=w272:u32)
        n96 = call <userlib>:"Tick Count (ms)__ogtk.vi"("error in (no error)"=w268) -> ("error out"=w276:errorcluster, "millisecond timer value"=w277:u32)  [unwired: 9 in]
        n97 = Subtract(x=w277, y=w272) -> (x-y=w274:u32)
        n98 = call <userlib>:"MGI Milliseconds Since Last Call.vi"("Error In"=w276) -> ("ms"=→"time b/w points (ms)":u32, "Error Out"=w267:errorcluster)  [unwired: 5 in]
        n99 = Divide(x=w274, y=u32 1000 ("x")) -> (x/y=→"elapsed time (s)":dbl)
        n100 = Bundle By Name(cluster=w270, "ms [i]"=w277) -> (w269:T8)
        n101 = call <vilib>:"Add State(s) to Queue__jki_lib_state_machine.vi"("State(s) in (\"\")"=w279) -> ("States Out"=w278:string)  [unwired: 14 in]
      }
      frame "---------- Macro ----------" {
        # "Do not put any code in this frame.\n(It is a separator no-op. You can make a copy of this frame to create a new Macro frame)"
        n102 = call <vilib>:"Add State(s) to Queue__jki_lib_state_machine.vi"("State(s) in (\"\")"=w283) -> ("States Out"=w282:string)  [unwired: 14 in]
      }
      frame "Macro: Initialize" {
        w284 = "Data: Initialize\nInitialize Core Data\nUI: Initialize\nUI: Front Panel State >> Open\nData: Initialize Top Level\nSweep: Initialize\nSweep: Start"  # Data: Initialize Initialize Core Data UI: Initialize UI: Front Panel State >> Open Data: Initialize Top Level Sweep: Initialize Sweep: Start
        # "Initialization Macro\n(This is called once, when the VI starts)"
        n103 = call <vilib>:"Add State(s) to Queue__jki_lib_state_machine.vi"("State(s) in Front (\"\")"=w284, "State(s) in (\"\")"=w288) -> ("States Out"=w287:string)  [unwired: 13 in]
      }
      frame "Macro: Sweep" {
        # "Initialization Macro\n(This is called once, when the VI starts)"
        n104 = call <vilib>:"Add State(s) to Queue__jki_lib_state_machine.vi"("State(s) in Front (\"\")"="Measure: Time\nMeasure: Lockin\nUI: Update Graphs\nUI: Update Timer", "State(s) in (\"\")"=w293) -> ("States Out"=w292:string)  [unwired: 13 in]
      }
      frame "Macro: Measure" {
        # "Initialization Macro\n(This is called once, when the VI starts)"
        n105 = call <vilib>:"Add State(s) to Queue__jki_lib_state_machine.vi"("State(s) in Front (\"\")"="Measure: Time\n//Measure: Temperature\n//Measure: Magnet\nMeasure: Lockin\nUI: Update Graphs", "State(s) in (\"\")"="", "State(s) at Back (\"\")"="Data: Check Notifier") -> ("States Out"=w296:string)  [unwired: 12 in]
        n106 = call <vilib>:"Add State(s) to Queue__jki_lib_state_machine.vi"("State(s) in Front (\"\")"=w296, "State(s) in (\"\")"=w301) -> ("States Out"=w300:string)  [unwired: 13 in]
      }
      frame "Macro: Exit" {
        # "Exit Macro\n(This is called once, when the VI exits)"
        n107 = Unbundle By Name(w308) -> ("Core.Close Panel on Exit?"=w307:bool)
        n108 = Select(t="UI: Front Panel State >> Close", s=w307, f="") -> (s? t:f=w304:string)
        n109 = call <vilib>:"Add State(s) to Queue__jki_lib_state_machine.vi"("State(s) in (\"\")"=w304, "State(s) at Back (\"\")"="Sweep: Stop\nFile: Save\nData: Cleanup\nExit") -> ("States Out"=w302:string)  [unwired: 13 in]
        n110 = call <vilib>:"Add State(s) to Queue__jki_lib_state_machine.vi"("State(s) in Front (\"\")"=w302, "State(s) in (\"\")"=w311) -> ("States Out"=w310:string)  [unwired: 13 in]
      }
      frame "---------- File ----------" {
        # "Template Separator\n(You can make a copy of, or modify, this frame)"
        n111 = call <vilib>:"Add State(s) to Queue__jki_lib_state_machine.vi"("State(s) in (\"\")"=w315) -> ("States Out"=w314:string)  [unwired: 14 in]
      }
      frame "File: Save" {
        # "Your code here.\n(You can make a copy of, or modify, this frame)"
        n112 = Unbundle By Name(w336) -> ("Execution:State"=w318:T9, "Control Experiment"=w332:refnum<class "SMO.Control Experiment.lvclass">, "AI Waveform (s)"=w333:waveform(dbl)[], "AO Waveform (s)"=w328:waveform(dbl)[])
        n113 = local read "Channels"() -> (w330:T1[])
        n114 = for {
          tunnel: w333 -> [w356] mode=indexing
          tunnel: w331 -> [w355]
          shift-right: [w340] -> w326
          shift-left: w332 -> [w351]
          tunnel: [w339] -> w327
          i -> [w348]
          n115 = call-poly <userlib>:"Waveform to XY.vi"("error in (no error)"=w355, "Waveform in"=w356) -> ("error out"=w357:errorcluster, "XY-data out"=w358:cluster{"X-array":dbl[], "Y-array":dbl[]})  [unwired: 8 in]
          n116 = Increment(x=w348) -> (x+1=w350:i32)
          n117 = call-poly <userlib>:"Get X and Y.vi"("error in (no error)"=w357, "XY-data"=w358) -> ("error out"=w342:errorcluster, "Y-array"=w343:dbl[], "X-array"=w344:dbl[])  [unwired: 6 in, 1 out]
          n118 = Format Into String(format string="Ch%d" ("wavenames"), w350) -> (resulting string=w347:string)  [unwired: 2 in, 1 out]
          n119 = Concatenate Strings(w347, "_x" ("string")) -> (w353:string)
          n120 = call "Write Dictionary Element.vi"("error in (no error)"=w342, "value"=w344, "key"=w353, "Control Experiment"=w351) -> ("error out"=w341:errorcluster, "Control Experiment out"=w352:refnum<class "SMO.Control Experiment.lvclass">)  [unwired: 6 in]
          n121 = Concatenate Strings(w347, "_y" ("string")) -> (w354:string)
          n122 = call "Write Dictionary Element.vi"("error in (no error)"=w341, "value"=w343, "key"=w354, "Control Experiment"=w352) -> ("error out"=w339:errorcluster, "Control Experiment out"=w340:refnum<class "SMO.Control Experiment.lvclass">)  [unwired: 6 in]
        }
        n123 = Index Array(array=w330) -> (element=w324:T1)  [unwired: 1 in]
        n124 = Unbundle By Name(w324) -> ("Channel"=w316:u16)
        n125 = Decrement(x=w316) -> (x-1=w329:u16)
        n126 = Format Into String(format string="Sweep %d" ("wavenames"), w316) -> (resulting string=w322:string)  [unwired: 2 in, 1 out]
        n127 = Index Array(array=w328, index=w329) -> (element=w321:waveform(dbl))
        n128 = Unbundle By Name(w321) -> ("Y"=w320:dbl[])
        n129 = call "Write Dictionary Element.vi"("error in (no error)"=w327, "value"=w320, "key"=w322, "Control Experiment"=w326) -> ("error out"=w325:errorcluster, "Control Experiment out"=w319:refnum<class "SMO.Control Experiment.lvclass">)  [unwired: 6 in]
        n130 = call "Exec State to Append.vi"("Execution:State"=w318) -> ("append?"=w317:bool)  [unwired: 2 in]
        n131 = call "Save Transport TDMS File.vi"("error in (no error)"=w325, "append?"=w317, "Control Experiment"=w319) -> ("error out"=w334:errorcluster)  [unwired: 7 in, 1 out]
        n132 = call <vilib>:"Clear Errors.vi"("error in (no error)"=w334) -> ("error out"=w335:errorcluster)  [unwired: 5 in, 1 out]
        n133 = call <vilib>:"Add State(s) to Queue__jki_lib_state_machine.vi"("State(s) in (\"\")"=w338) -> ("States Out"=w337:string)  [unwired: 14 in]
      }
      frame "---------- Sweep ----------" {
        # "Template Separator\n(You can make a copy of, or modify, this frame)"
        n134 = call <vilib>:"Add State(s) to Queue__jki_lib_state_machine.vi"("State(s) in (\"\")"=w362) -> ("States Out"=w361:string)  [unwired: 14 in]
      }
      frame "Sweep: Initialize" {
        # "Template Separator\n(You can make a copy of, or modify, this frame)"
        n135 = Unbundle By Name(w372) -> ("Instruments.Lockin"=w371:refnum<class "Instrument.Lockin.lvclass">)
        n136 = Bundle By Name(cluster=T7 {"Sweep Time (s)"=0.0, "Initial Wait (s)"=0.0, "Return to Start"=FALSE, "Channels"=[]} ("Configure Sweep"), "Sweep Time (s)"="Sweep Time (s)", "Initial Wait (s)"="Initial Wait (s)", "Return to Start"="Return to Start", "Channels"="Channels") -> (w367:T7)
        n137 = call <userlib>:"setSweepConfiguration.vi"("error in (no error)"=w370, "Configure Sweep"=w367, "Instrument.Lockin in"=w371) -> ("error out"=w369:errorcluster)  [unwired: 7 in, 1 out]
        n138 = call <vilib>:"Add State(s) to Queue__jki_lib_state_machine.vi"("State(s) in (\"\")"=w374) -> ("States Out"=w373:string)  [unwired: 14 in]
      }
      frame "Sweep: Start" {
        # "wait for sweeping to start"
        # "Template Separator\n(You can make a copy of, or modify, this frame)"
        n139 = Unbundle By Name(w377) -> ("Instruments.Lockin"=w378:refnum<class "Instrument.Lockin.lvclass">)
        n140 = call <userlib>:"startSweep.vi"("error in (no error)"=w376, "Instrument.Lockin in"=w378) -> ("error out"=w380:errorcluster, "Instrument.Lockin out"=w379:refnum<class "Instrument.Lockin.lvclass">)  [unwired: 8 in]
        n141 = while {
          shift-right: [w390] -> w375
          shift-left: w380 -> [w391]
          tunnel: w379 -> [w387]
          tunnel: [w386] -> _
          stop <- w388 stop-if-true
          n142 = call <userlib>:"Wait (ms)__ogtk.vi"("error in (no error)"=w391, "milliseconds to wait"=u32 1000) -> ("error out"=w385:errorcluster)  [unwired: 8 in, 1 out]
          n143 = call <userlib>:"getStatus.vi"("error in (no error)"=w385, "Instrument.Lockin"=w387) -> ("error out"=w390:errorcluster, "Status"=w389:T11, "Instrument.Lockin"=w386:refnum<class "Instrument.Lockin.lvclass">)  [unwired: 7 in]
          n144 = Equal?(x=State-enum."sweeping" ("Status 2"), y=w389) -> (x = y?=w388:bool)
        }
        n145 = call <vilib>:"Add State(s) to Queue__jki_lib_state_machine.vi"("State(s) in (\"\")"=w382) -> ("States Out"=w381:string)  [unwired: 14 in]
      }
      frame "Sweep: Stop" {
        # "Template Separator\n(You can make a copy of, or modify, this frame)"
        n146 = Unbundle By Name(w394) -> ("Instruments.Lockin"=w395:refnum<class "Instrument.Lockin.lvclass">)
        n147 = call <userlib>:"stopSweep.vi"("error in (no error)"=w393, "Instrument.Lockin in"=w395) -> ("error out"=w392:errorcluster)  [unwired: 8 in, 1 out]
        n148 = call <vilib>:"Add State(s) to Queue__jki_lib_state_machine.vi"("State(s) in (\"\")"=w397) -> ("States Out"=w396:string)  [unwired: 14 in]
      }
      frame "Sweep: Check State" {
        # "Template Separator\n(You can make a copy of, or modify, this frame)"
        n149 = Unbundle By Name(w398) -> ("Instruments.Lockin"=w402:refnum<class "Instrument.Lockin.lvclass">)
        n150 = call <userlib>:"getStatus.vi"("error in (no error)"=w401, "Instrument.Lockin"=w402) -> ("error out"=w400:errorcluster, "Status"=w403:T11)  [unwired: 7 in, 1 out]
        "Status" <- w403
        n151 = case shown="Default" w403 {
          tunnel: ["Macro: Exit" ("State(s) in Front (\"\")") "Macro: Sweep" ("State(s) in Front (\"\")")] -> w399
          frame Default {
          }
          frame "sweeping" {
          }
        }
        n152 = call <vilib>:"Add State(s) to Queue__jki_lib_state_machine.vi"("State(s) in Front (\"\")"=w399, "State(s) in (\"\")"=w405) -> ("States Out"=w404:string)  [unwired: 13 in]
      }
      frame "---------- Measure ----------" {
        # "Do not put any code in this frame.\n(It is a separator no-op. You can make a copy of this frame to create a new Macro frame)"
        n153 = call <vilib>:"Add State(s) to Queue__jki_lib_state_machine.vi"("State(s) in (\"\")"=w411) -> ("States Out"=w410:string)  [unwired: 14 in]
      }
      frame "Measure: Time" {
        # "Do not put any code in this frame.\n(It is a separator no-op. You can make a copy of this frame to create a new Macro frame)"
        n154 = Unbundle By Name(w418) -> ("Control Experiment"=w417:refnum<class "SMO.Control Experiment.lvclass">)
        n155 = Get Date/Time In Seconds() -> (seconds since 1Jan1904=w420:timestamp)
        n156 = To Double Precision Float(number=w420) -> (double precision float=w413:dbl)
        n157 = call "Append Dictionary Element.vi"("error in (no error)"=w415, "value"=w413, "key"="Time", "Control Experiment"=w417) -> ("error out"=w412:errorcluster, "Control Experiment out"=w416:refnum<class "SMO.Control Experiment.lvclass">)  [unwired: 6 in]
        n158 = Bundle By Name(cluster=w418, "Control Experiment"=w416) -> (w419:T8)
        n159 = call <vilib>:"Add State(s) to Queue__jki_lib_state_machine.vi"("State(s) in (\"\")"=w422) -> ("States Out"=w421:string)  [unwired: 14 in]
      }
      frame "Measure: Temperature" {
        # "Do not put any code in this frame.\n(It is a separator no-op. You can make a copy of this frame to create a new Macro frame)"
        n160 = Unbundle By Name(w430) -> ("Control Experiment"=w425:refnum<class "SMO.Control Experiment.lvclass">, "Instruments.Temperature"=w432:refnum<class "Instrument.Cryostat.lvclass">)
        n161 = call-dynamic "Get Temperature.vi"("error in (no error)"=w431, "Instrument.Cryostat in"=w432) -> ("error out"=w426:errorcluster, "Temperature (K)"=w427:dbl)  [unwired: 5 in, 3 out]
        n162 = call "Append Dictionary Element.vi"("error in (no error)"=w426, "value"=w427, "key"="Temperature", "Control Experiment"=w425) -> ("error out"=w423:errorcluster, "Control Experiment out"=w424:refnum<class "SMO.Control Experiment.lvclass">)  [unwired: 6 in]
        n163 = Bundle By Name(cluster=w430, "Control Experiment"=w424) -> (w429:T8)
        n164 = call <vilib>:"Add State(s) to Queue__jki_lib_state_machine.vi"("State(s) in (\"\")"=w434) -> ("States Out"=w433:string)  [unwired: 14 in]
      }
      frame "Measure: Magnet" {
        # "Do not put any code in this frame.\n(It is a separator no-op. You can make a copy of this frame to create a new Macro frame)"
        n165 = Unbundle By Name(w444) -> ("Control Experiment"=w441:refnum<class "SMO.Control Experiment.lvclass">, "Instruments.Temperature"=w436:refnum<class "Instrument.Cryostat.lvclass">)
        n166 = call-dynamic "Get Magnet Field.vi"("error in (no error)"=w438, "Instrument.Cryostat in"=w436) -> ("error out"=w437:errorcluster, "B Field (T)"=w435:dbl)  [unwired: 5 in, 3 out]
        n167 = call "Append Dictionary Element.vi"("error in (no error)"=w437, "value"=w435, "key"="Magnet", "Control Experiment"=w441) -> ("error out"=w439:errorcluster, "Control Experiment out"=w440:refnum<class "SMO.Control Experiment.lvclass">)  [unwired: 6 in]
        n168 = Bundle By Name(cluster=w444, "Control Experiment"=w440) -> (w443:T8)
        n169 = call <vilib>:"Add State(s) to Queue__jki_lib_state_machine.vi"("State(s) in (\"\")"=w446) -> ("States Out"=w445:string)  [unwired: 14 in]
      }
      frame "Measure: Lockin" {
        # "Do not put any code in this frame.\n(It is a separator no-op. You can make a copy of this frame to create a new Macro frame)"
        n170 = Unbundle By Name(w457) -> ("t0"=w454:timestamp, "AI Waveform (s)"=w450:waveform(dbl)[], "Instruments.Lockin"=w453:refnum<class "Instrument.Lockin.lvclass">, "AO Waveform (s)"=w447:waveform(dbl)[])
        n171 = Array Size(array=w450) -> (size(s)=w449:i32)
        n172 = case shown="0" w449 {
          tunnel: w450 -> [_ w489]
          tunnel: [w464 w488] -> w456
          tunnel: [w463 w487] -> w451
          tunnel: w452 -> [w468 w486]
          tunnel: [w465 w482] -> w455
          tunnel: w453 -> [w469 w481]
          tunnel: w454 -> [_ w479]
          tunnel: [w461 w475] -> w448
          tunnel: w447 -> [_ w476]
          frame 0 {
            n173 = for {
              N: 3 -> [_]
              tunnel: w469 -> [w474]
              tunnel: [w472] -> w464
              tunnel: w468 -> [w473]
              tunnel: [w471] -> w463
              tunnel: [w470] -> w462
              n174 = call <userlib>:"waitForNewWaveforms.vi"("error in (no error)"=w473, "Instrument.Lockin in"=w474) -> ("error out"=w471:errorcluster, "Newest AI Waveform"=w472:waveform(dbl)[], "Instrument.Lockin out"=w470:refnum<class "Instrument.Lockin.lvclass">)  [unwired: 7 in]
            }
            n175 = Index Array(array=w464) -> (element=w467:waveform(dbl))  [unwired: 1 in]
            n176 = Unbundle By Name(w467) -> ("t0"=w465:timestamp)
            n177 = call <userlib>:"getAO.vi"("error in (no error)"=w463, "Instrument.Lockin in"=w462) -> ("AOconfig"=w461:T12)  [unwired: 7 in, 2 out]
          }
          frame Default {
            n178 = call <userlib>:"getAI.vi"("error in (no error)"=w486, "Instrument.Lockin in"=w481) -> ("error out"=w485:errorcluster, "AI Waveform"=w480:waveform(dbl)[], "Instrument.Lockin out"=w478:refnum<class "Instrument.Lockin.lvclass">)  [unwired: 7 in]
            n179 = Index Array(array=w480) -> (element=w484:waveform(dbl))  [unwired: 1 in]
            n180 = call <userlib>:"getAO.vi"("Instrument.Lockin in"=w478) -> ("AOconfig"=w477:T12)  [unwired: 8 in, 2 out]
            n181 = Unbundle By Name(w484) -> ("t0"=w482:timestamp)
            n182 = Equal?(x=w482, y=w479) -> (x = y?=w483:bool)
            n183 = case shown="True" w483 {
              tunnel: w489 -> [w494 w521]
              tunnel: [w497 w521] -> w488
              tunnel: [w496 w522] -> w487
              tunnel: w485 -> [w495 w522]
              tunnel: w480 -> [w498 _]
              tunnel: w477 -> [w492 _]
              tunnel: w476 -> [w491 w520]
              tunnel: [w490 w520] -> w475
              frame False {
                n184 = Array Size(array=w494) -> (size(s)=w493:i32)
                n185 = case shown="0" w493 {
                  tunnel: w498 -> [w501 w509]
                  tunnel: [w501 w508] -> w497
                  tunnel: [w500 w507] -> w496
                  tunnel: w495 -> [w500 w503]
                  tunnel: w494 -> [_ w506]
                  tunnel: w492 -> [_ w505]
                  tunnel: w491 -> [w499 w504]
                  tunnel: [w499 w502] -> w490
                  frame 0 {
                  }
                  frame Default {
                    n186 = for {
                      tunnel: w506 -> [w515] mode=indexing
                      tunnel: w509 -> [w519] mode=indexing
                      tunnel: [w518] -> w508 mode=indexing
                      tunnel: [w517] -> w507
                      tunnel: w503 -> [w516]
                      n187 = call-poly <vilib>:"Append Waveforms.vi"("error in (no error)"=w516, "waveform B"=w519, "waveform A"=w515) -> ("error out"=w517:errorcluster, "waveform out"=w518:waveform(dbl))  [unwired: 7 in]
                    }
                    n188 = for {
                      tunnel: w504 -> [w510] mode=indexing
                      tunnel: w505 -> [w514] mode=indexing
                      tunnel: [w513] -> w502 mode=indexing
                      tunnel: [w512] -> _
                      tunnel: w503 -> [w511]
                      n189 = call-poly <vilib>:"Append Waveforms.vi"("error in (no error)"=w511, "waveform B"=w514, "waveform A"=w510) -> ("error out"=w512:errorcluster, "waveform out"=w513:waveform(dbl))  [unwired: 7 in]
                    }
                  }
                }
              }
              frame True {
              }
            }
          }
        }
        n190 = Bundle By Name(cluster=w457, "t0"=w455, "AI Waveform (s)"=w456, "AO Waveform (s)"=w448) -> (w458:T8)
        n191 = call <vilib>:"Add State(s) to Queue__jki_lib_state_machine.vi"("State(s) in (\"\")"=w460) -> ("States Out"=w459:string)  [unwired: 14 in]
      }
    }
  }
  "error out" <- w3
  n192 = Unbundle By Name(w2) -> ("Transport"=→"Transport.lvclass":refnum<class "SMO.Transport.lvclass">)
